vi "HomeMove.vi"(11 "UiDefinition":T1) -> ()   [LabVIEW 2020]
uses:
  UIReferences.ctl
  D:/LabviewDXFViewer/LabviewDXFViewer/bin/Release/LabviewDXFViewer.exe
  LabviewDXFViewer/bin/Release/LabviewDXFViewer.exe
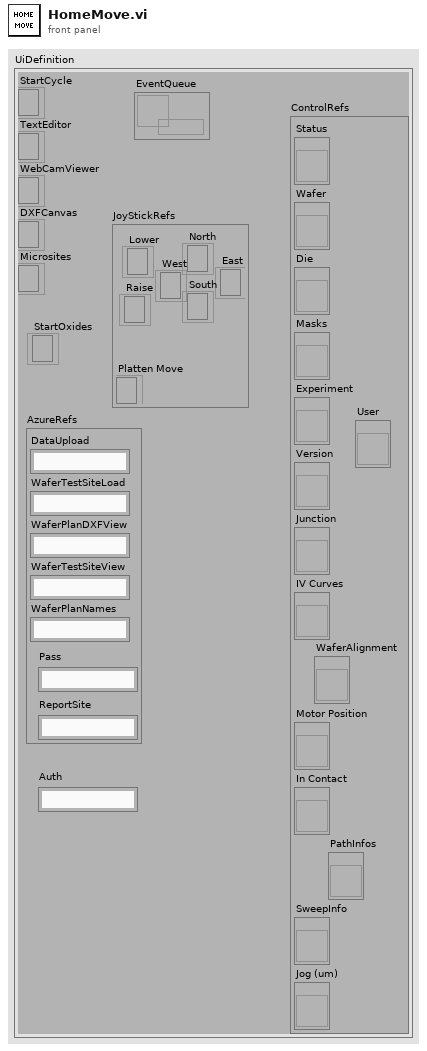
[diagram p1: front panel]
types:
  T1 = typedef "UIReferences.ctl" = cluster{"StartCycle":refnum<k24>, "TextEditor":refnum<k24>, "WebCamViewer":refnum<k24>, "DXFCanvas":refnum<k24>, "Microsites":refnum<k24>, "JoyStickRefs":cluster{"North":refnum<k24>, "Lower":refnum<k24>, "Raise":refnum<k24>, "Platten Move":refnum<k24>, "West":refnum<k24>, "East":refnum<k24>, "South":refnum<k24>}, "AzureRefs":cluster{"DataUpload":string, "WaferTestSiteLoad":string, "WaferPlanDXFView":string, "WaferTestSiteView":string, "WaferPlanNames":string, "Pass":string, "ReportSite":string}, "ControlRefs":cluster{"Status":refnum<vi>, "Wafer":refnum<vi>, "Die":refnum<vi>, "Masks":refnum<vi>, "Experiment":refnum<vi>, "Version":refnum<vi>, "Junction":refnum<vi>, "IV Curves":refnum<vi>, "Motor Position":refnum<vi>, "In Contact":refnum<vi>, "SweepInfo":refnum<vi>, "Jog (um)":refnum<vi>, "PathInfos":refnum<vi>, "User":refnum<vi>, "WaferAlignment":refnum<vi>}, "EventQueue":refnum<queue>, "StartOxides":refnum<k24>, "Auth":string}
  T2 = typedef "WaferAlignmentType.ctl" = cluster{"Wafer Units to microns":dbl, "Rotation Misalign":dbl[], "Scale Misalign":dbl, "Steps Per micron":dbl, "Position 1":i32[], "Position 2":i32[], "Lift Distance":i32, "Position 3":i32[], "Jog Height":i32}
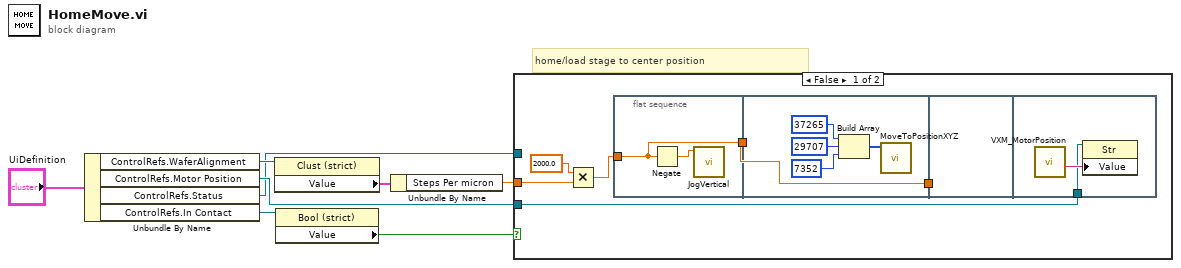
[diagram p0: block diagram]
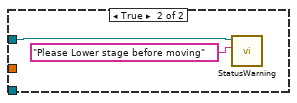
[diagram p2: hidden frame]
diagram:
  # "home/load stage to center position"
  n1 = Unbundle By Name("UiDefinition") -> ("ControlRefs.WaferAlignment"=w6:refnum<vi>, "ControlRefs.Motor Position"=w4:refnum<vi>, "ControlRefs.Status"=w3:refnum<vi>, "ControlRefs.In Contact"=w2:refnum<vi>)
  n2 = property class="Clust (strict)"(reference=w6) -> ("Value"=w5:T2)  [unwired: 1 in, 2 out]
  n3 = property class="Bool (strict)"(reference=w2) -> ("Value"=w1:bool)  [unwired: 1 in, 2 out]
  n4 = Unbundle By Name(w5) -> ("Steps Per micron"=w8:dbl)
  n5 = case shown="False" w1 {
    tunnel: w3 -> [_ w24]
    tunnel: w8 -> [w12 _]
    tunnel: w4 -> [w10 _]
    frame False {
      n6 = Multiply(x=2000.0, y=w12) -> (x*y=w11:dbl)
      n7 = flat-sequence {
        tunnel: [w15] -> w13
        tunnel: w11 -> [w15]
        tunnel: [w21] -> w14
        tunnel: w13 -> [w21]
        tunnel: w14 -> [_]
        tunnel: w10 -> [w22]
        frame #0 {
          n8 = Negate(x=w15) -> (-x=w16:dbl)
          n9 = call "JogVertical.vi"("Numeric"=w16) -> ()  [unwired: 11 in]
        }
        frame #1 {
          n10 = Build Array(37265 ("X"), 29707 ("Y"), 7352 ("Y")) -> (w17:i32[])
          n11 = call "MoveToPositionXYZ.vi"("Array"=w17) -> ()  [unwired: 11 in]
        }
        frame #2 {
        }
        frame #3 {
          n12 = call "VXM_MotorPosition.vi"() -> ("Position String"=w23:string)  [unwired: 10 in, 1 out]
          n13 = property class="Str"(reference=w22, "Value"=w23) -> ()  [unwired: 1 in, 2 out]
        }
      }
    }
    frame True {
      n14 = call "StatusWarning.vi"("Text.Text"="Please Lower stage before moving" ("Status"), "String in"=w24) -> ()  [unwired: 10 in]
    }
  }
